vi "PH_TKTDS-30xx.Close.vi"(0 "i ref in":refnum<vi>, 5 "error in(no error)":errorcluster) -> (14 "i ref out":refnum<vi>, 19 "error out":errorcluster)   [LabVIEW 2014, in "PH_TKTDS-30xx.lvlib"]
doc: "This VI closes the connection and sets the connection established and the error flag at own attributes to false."
uses:
  PH_TKTDS-30xx.lvlib
  PH_Basics/PH_StatusHandler/PH_StatusHandler.Status.ctl
  instr.lib/TKDS3032-PHELIX/tktds3032-PHELIX - Driver np.lvlib
  PH_Basics/PH_StatusHandler/PH_StatusHandler.lvlib
  PH_Basics/PH_Common/PH_Common.lvlib
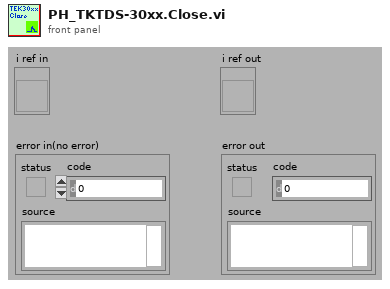
[diagram p1: front panel]
types:
  T1 = typedef "PH_TKTDS-30xx.lvlib/PH_TKTDS-30xx.i attribute.ctl" = cluster{"Default VISA Resource":string, "VISA Resource Name":refnum<visa-resource-name>, "Revision":cluster{"Instrument Driver":string, "Instrument Firmware":string}, "Selftest":cluster{"Result":u32, "Message":string}, "Channels":T2[], "Trigger Configuration":T4, "Acquisition Configuration":T5, "Fetched Waveforms":T6[], "GUI Refs":T7, "State":T8, "Error Message":string, "Allow Prdc Loop?":bool}
  T2 = typedef "PH_TKTDS-30xx.lvlib/PH_TKTDS-30xx.Channel Config.ctl" = cluster{"Channel Name":string, "Input Impedance":string, "Max Input Frequency":string, "Vertical Coupling":i32, "Channel Enabled":bool, "Probe Attenuation":dbl, "Vertical Range":dbl, "Vertical Offset":dbl, "Waveform Limits":T3}
  T3 = typedef "PH_TKTDS-30xx.lvlib/PH_TKTDS-30xx.Waveform Limits.ctl" = cluster{"Start":i32, "End":i32}
  T4 = typedef "PH_TKTDS-30xx.lvlib/PH_TKTDS-30xx.Trigger Config.ctl" = cluster{"Source":string, "Slope":i32, "Level [V]":dbl}
  T5 = typedef "PH_TKTDS-30xx.lvlib/PH_TKTDS-30xx.Acquisition Config.ctl" = cluster{"Time base":dbl, "Record Length":u16, "Start Time":dbl, "Type":i32, "Continuous":bool}
  T6 = typedef "PH_TKTDS-30xx.lvlib/PH_TKTDS-30xx.fetched Waveform.ctl" = cluster{"Source":string, "Actual Points":u32, "Initial X":dbl, "X Increment":dbl, "Waveform Array":dbl[]}
  T7 = typedef "PH_TKTDS-30xx.lvlib/PH_TKTDS-30xx.GUI Refs.ctl" = cluster{"Trigger":refnum<vi>, "Acquisition":refnum<vi>, "State":refnum<vi>, "Delete":refnum<vi>, "Channel to be positioned":refnum<vi>, "Postion":refnum<vi>, "Display Intensity":refnum<vi>, "VISA Resource":refnum<vi>, "Channels":refnum<vi>[], "Graphs":refnum<vi>[]}
  T8 = typedef "PH_StatusHandler.lvlib/PH_StatusHandler.Status.ctl" = i16
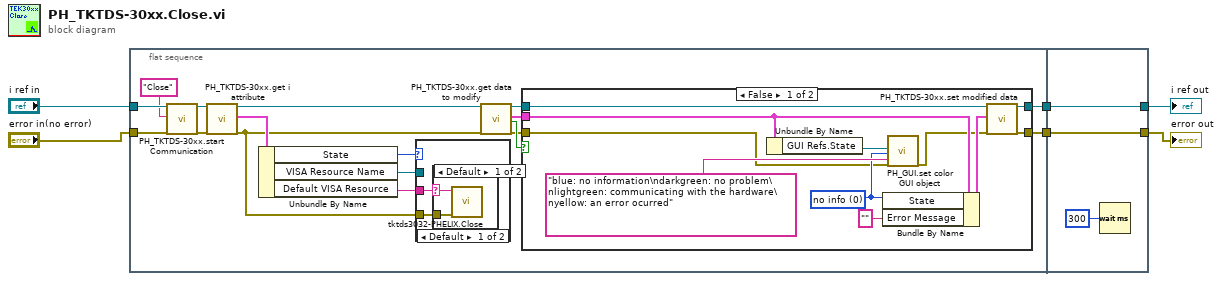
[diagram p0: block diagram]
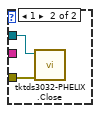
[diagram p3: hidden frame]
diagram:
  n1 = flat-sequence {
    tunnel: "error in(no error)" -> [w22]
    tunnel: "i ref in" -> [w9]
    tunnel: [w19] -> w2
    tunnel: [w18] -> w1
    tunnel: [w44] -> w4
    tunnel: [w45] -> w5
    tunnel: w2 -> [w45]
    tunnel: w1 -> [w44]
    frame #0 {
      n2 = call "PH_TKTDS-30xx.start Communication.vi"("i ref in"=w9, "Action"="Close", "error in"=w22) -> ("i ref out"=w8:refnum<vi>, "error out"=w10:errorcluster)  [unwired: 15 in]
      n3 = call "PH_TKTDS-30xx.get i attribute.vi"("i ref in"=w8, "error in (no error)"=w10) -> ("i ref out"=w20:refnum<vi>, "i attribute"=w23:T1, "error out"=w12:errorcluster)  [unwired: 15 in]
      n4 = Unbundle By Name(w23) -> ("State"=w13:T8, "VISA Resource Name"=w14:refnum<visa-resource-name>, "Default VISA Resource"=w11:string)
      n5 = case shown="Default" w13 {
        tunnel: w14 -> [_ w29]
        tunnel: w12 -> [w24 w28]
        tunnel: w11 -> [w25 _]
        frame Default {
          n6 = case shown="Default" w25 {
            selector: w25 -> [w27 _]
            tunnel: w24 -> [w26 _]
            frame Default {
              n7 = call "tktds3032-PHELIX.Close.vi"("error in (no error)"=w26, "VISA Resource Name"=w27) -> ()  [unwired: 9 in, 1 out]
            }
            frame "", "N/A" {
            }
          }
        }
        frame 1 {
          n8 = call "tktds3032-PHELIX.Close.vi"("error in (no error)"=w28, "VISA Resource Name"=w29) -> ()  [unwired: 9 in, 1 out]
        }
      }
      n9 = call "PH_TKTDS-30xx.get data to modify.vi"("i ref in"=w20, "error in (no error)"=w12) -> ("i ref out"=w17:refnum<vi>, "i attribute"=w16:T1, "timed out"=w21:bool, "error out"=w15:errorcluster)  [unwired: 14 in]
      n10 = case shown="False" w21 {
        tunnel: [w40 w41] -> w18
        tunnel: w15 -> [w31 w41]
        tunnel: w17 -> [w39 w42]
        tunnel: [w38 w42] -> w19
        tunnel: w16 -> [w35 _]
        frame False {
          w32 = T8 0 items=["no info", "off/false/out", "on/true/in", "Failure", "Alarm", "Status 1", "Status 2", "Status 3"] ("State")
          n11 = Unbundle By Name(w35) -> ("GUI Refs.State"=w34:refnum<vi>)
          n12 = Bundle By Name(cluster=w35, "State"=w32, "Error Message"="" ("Error.Message")) -> (w37:T1)
          n13 = call "PH_GUI.set color GUI object.vi"("GUI object Ref"=w34, "State"=w32, "error in (no error)"=w31, "Tip Strip (N/A)"="blue: no information\ndarkgreen: no problem\nlightgreen: communicating with the hardware\nyellow: an error ocurred") -> ("error out"=w30:errorcluster)  [unwired: 15 in]
          n14 = call "PH_TKTDS-30xx.set modified data.vi"("i ref in"=w39, "i attribute"=w37, "error in (no error)"=w30) -> ("i ref out"=w38:refnum<vi>, "error out"=w40:errorcluster)  [unwired: 15 in]
        }
        frame True {
        }
      }
    }
    frame #1 {
      n15 = Wait (ms)(milliseconds to wait=u32 300) -> ()  [unwired: 1 out]
    }
  }
  "error out" <- w4
  "i ref out" <- w5
